vi "Big_LED_control.vi"() -> ()   [LabVIEW 2018]
uses:
  C:/Users/user/Desktop/LabVIEW/LED_CONTROL_big/LED_CONTROL_big_LED_ophir_ready/AT lib/AmateurStepperMotor.dll
  AT lib/AmateurStepperMotor.dll
  <instrlib>/niDMM/nidmm.llb/niDMM Function.ctl
  <instrlib>/niDMM/nidmm.llb/niDMM Resolution in Digits.ctl
  <instrlib>/niDCPower/nidcpower.llb/niDCPower Measurement Type.ctl
  <vilib>/Instr/_visa.llb/VISA Configure Serial Port (Instr).vi
  <instrlib>/niDMM/nidmm.llb/niDMM Configure Measurement Digits.vi
panel:
  in  "Tab Control 2":enum32{"Шаговик и офир", "Служебная область"}(tab)
  in  "milliseconds to wait":u32=1000
  in  "Go To":dbl
  out "Ophir 1 Char":dbl(graph)=0.060000000000000005
  in  "DecelerationTime, s":dbl
  in  "AccelerationTime, s":dbl
  in  "HoldOn":bool
  in  "Ophir 1 units":string(combo)="1000" caption="Units"
  out "Ophir 1 Over Range":bool caption="Over Range"
  out "Ophir 1 Optical Power":dbl=0.060000000000000005 caption="Power" format="%#_4g"
  out "Ophir 1 MAX":dbl=0.060000000000000005 caption="MAX" format="%#_5g"
  in  "Ophir 1 Clear":bool caption="Clear"
  in  "StepMultiplicationFactor":dbl=1.0
  in  "StepDivisor":i32(ring)=8 items=["D1"=1, "D2"=2, "D4"=4, "D8"=8, "D16"=16, "D32"=32]
  in  "Speed":dbl=1000.0
  in  "Погнали!":bool
  in  "Стоп GoTo":bool
  out "Готово":bool
  out "Position":dbl
  in  "Ophir 1 Info":u16(ring)=1 caption="Info" items=["Device : JUNO; s/n:903793", "Head : PD300R-3W   ; s/n:779628"]
  in  "new pos":dbl
  in  "set pos":bool
  out "Device Response":string="*\n"
  in  "Ophir 1 usb channel":i16 caption="usb channel"
  out "Ophir 1 dup Visa Session":refnum<visa-resource-name>="USB0::0x0BD3::0x0777::NI-VISA-40004::RAW" caption="dup Visa Session"
  in  "Ophir 1 Baud Rate (3:9600)":i16(ring)=3 caption="Baud Rate (3:9600)" items=["300", "1200", "4800", "9600", "19200", "38400"]
  out "Ophir 1 Real Optical Power":dbl=6e-05 format="%.6e"
  in  "Ophir 1 GPIB Address (10)":string="10" caption="GPIB Address (10)"
  in  "Ophir 1 Port Number (default 2)":i16=1 caption="Port Number (default 2)" min=0 max=20
  in  "Ophir 1 Select Communication Protocol":u16(ring) caption="Select Communication Protocol" items=["USB", "RS232", "GPIB"]
  out "Ophir 1 error out":errorcluster caption="error out"
  in  "Ophir 1 error in (no error)":errorcluster caption="error in (no error)"
  in  "Ophir 1 Wait":u32=100 caption="Wait"
  out "IsOpen":bool
  out "Ophir 1 Initialization":bool=TRUE caption="Initialization"
  in  "Tab Control":T1(tab)=enum."Служебная область"
  in  "POWER":bool
  in  "Стоп":bool=TRUE
  in  "Resource Name":refnum<k15>="PXI1Slot2" caption="Источник питания"
  in  "Амперметр":refnum<k15>="PXI1Slot4" caption="NI DMM 1"
  in  "V_MB, V":dbl=5.0 caption="voltage level" format="%_6p"
  in  "curlim_V_MB, A":dbl=0.3 caption="current limit" format="%_6p"
  out "curmes_V_MB, A":dbl=-0.001986406197333734 caption="measurement" format="%_6g"
  out "chart_0":dbl(graph)=-0.001986406197333734 caption="Waveform Chart 5"
  in  "voltlim_I_LED, V":dbl=0.01 caption="current limit" min=0.01 format="%_6p"
  in  "I_LED, A":dbl=2.000000000000001 caption="voltage level" format="%_6p"
  out "chart_1":dbl(graph)=9.464711192498274e-07 caption="Waveform Chart 5"
  out "voltmes_V_LED, A":dbl=9.464711192498274e-07 caption="measurement" format="%_6g"
  out "Current Char":dbl(graph)=0.008323229849338531
  in  "Arduino":refnum<visa-resource-name>="COM14"
  in  "Сегменты":bool[](array[boolean])=[FALSE, FALSE, FALSE, FALSE, FALSE, FALSE, FALSE, FALSE, FALSE, FALSE, FALSE, FALSE, FALSE, FALSE, FALSE, FALSE, FALSE, FALSE]
  in  "Вольтметр":refnum<k15>="PXI1Slot5" caption="NI DMM 1"
  out "Voltage Char":dbl(graph)=nan
  in  "Port Name":string="COM1" caption="Порт шаговика"
  in  "wave_lenght":string="600"
  in  "Промер":bool caption="Промер сегмента"
  in  "NI DMM 1 Voltage Range 4":string(combo)="-1" caption="Range"
  in  "NI DMM 1 units 4":string(combo)="1" caption="Units"
  out "Voltage":dbl=nan format="%_6g"
  in  "NI DMM 1 Current Range 3":string(combo)="1" caption="Range"
  in  "NI DMM 1 units 3":string(combo)="1000" caption="Units"
  out "Current":dbl=0.008323229849338531 format="%_6g"
  out "Разряд":dbl
  out "+/-":bool
  out "Power off":bool=TRUE
  in  "Command":string="Anode"
  in  "Записать":bool
  out "measure output file refnum":refnum<file>
  out "Voltage, V":dbl=nan caption="Measurement" format="%.5f"
  out "Current, A":dbl=8.323229849338531e-06 caption="Measurement" format="%.5f"
  out "Тип индикатора":string="Anode"
  out "chart_2":dbl(graph)=4.286668577189643e-07
  in  "V_RES, V":dbl caption="voltage level" format="%_6p"
  out "curmes_V_RES, A":dbl=4.286668577189643e-07 caption="measurement" format="%_6g"
  in  "curlim_V_RES, A":dbl=0.1 caption="current limit" min=0.01 format="%_6p"
  in  "measure path":path=path "D:/NI LabVIEW/MultiOpto/MultiOpto_1.2/Logs/SEL"
  out "Enum":enum16{"Exit", "4", "Промер", "2", "1"}(ring)
  out "№ об-ца":dbl
  out "Темп-ра":dbl
  out "Сегмент":string
  # "Шаговик"
  # "Офир"
  # "Шаговик"
  # "Офир"
  # "position - это значение абсолютное"
  # "j"
  # "c"
  # "d"
  # "e"
  # "g"
  # "h"
  # "a"
  # "b"
  # "f"
  # "k"
  # "L"
  # "m"
  # "n"
  # "p"
  # "dp"
  # "all"
  # "V_MB 5 В\nогрничение 300 м\n\nV_LED 2,1 В\nограничение 200 м"
  # "единицы мА\nrange 1 А"
  # "1. каждый сегмент включаем по отдельности, резистором постраиваем ток до 10 мА\n2. напряжение V_LED при этом не меняется\n3. в такоом положении промеряем сегменты по отдельности\n4. для промера всего индикатора сразу подстраиваем напряжение при неизменном положении резисторов\n5. ток всех индикаторов = ток одного сегмента (10 мА) * число сегментов (15)\n6. добиваемся этого увеличением V_LED"
  # "единицы В\nrange AUTO"
  # "регклировка суммарного тока через индикатор"
  # "24.063\n\n     I          U\n20 мА  1.3 В\n20 мА  1.4 В\n 7 мА   1.15 В"
  # "24.064\n\n     I          U\n10 мА  2 В\n10 мА  2.15 В\n 7 мА   1.9 В"
  # "автоматизировать подбор напряжения по известному максимальному напряжению и току. ОС по току сегмента"
  # "Р1:  +25°C\nР2:  - 60°C\nР3:  +85°C"
  # "регулировать ток в зависимости от температуры.\nс ростом температуры растет ток.\nпид-регулятор??"
  # "0. ввести номер образца\n1. включить нужный сегмент\n2. ввести его в поле справа\n3. вести температуру в поле слева\n4. нажать кнопку \"промер сегмента\""
  # "\"опрашивать кнопки не чаще, чем раз в секунду. сейчас кликать можно чаще, они загорятся, но ничего не произойдет\""
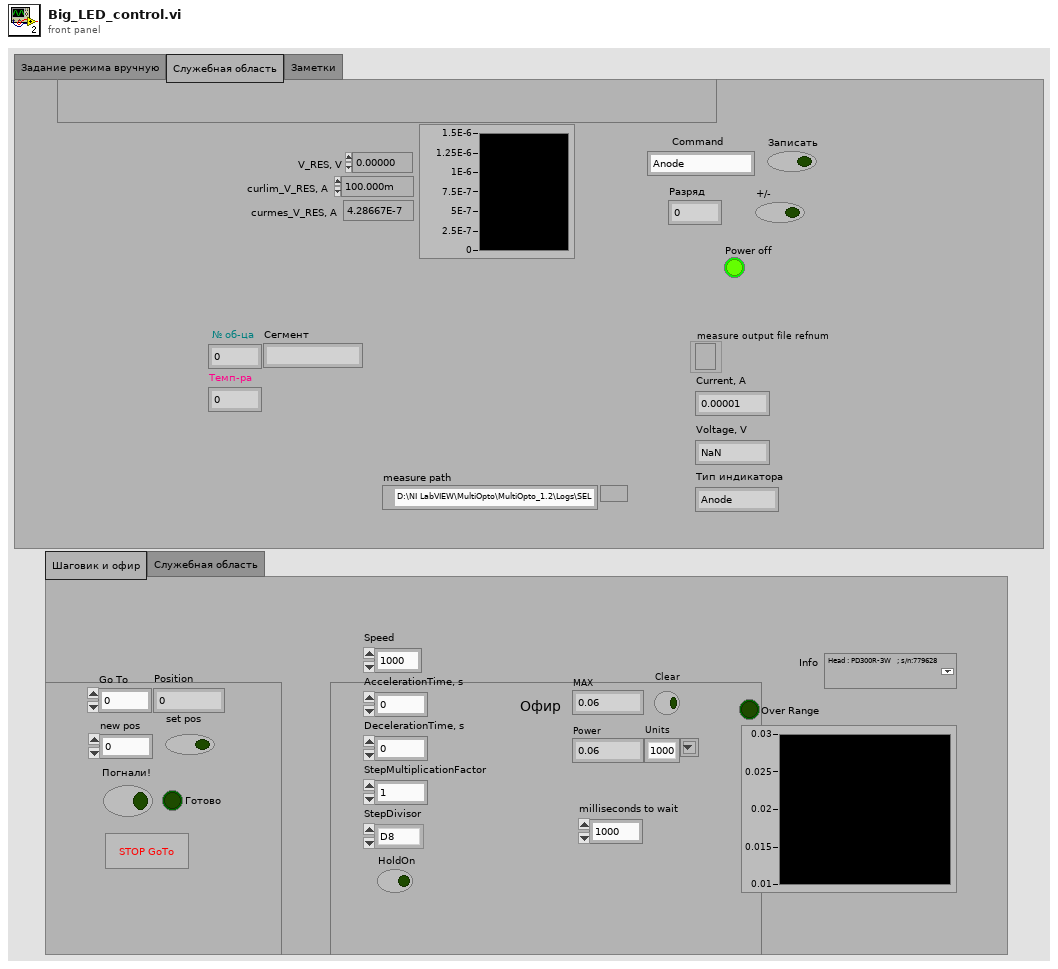
[diagram p1: front panel]
types:
  T1 = enum32{"Задание режима вручную", "Служебная область", "Заметки"}
  T2 = enum16{"open", "replace", "create", "open or create", "replace or create", "replace or create with confirmation"}
  T3 = typedef "niDCPower Measurement Type.ctl" = i32
  T4 = typedef "niDMM Function.ctl" = enum16{"DC Volts", "AC Volts", "DC Current", "AC Current", "2-wire Resistance", "4-wire Resistance", "Diode", "Frequency", "Period", "AC Volts DC Coupled", "Capacitance", "Inductance", "Temperature"}
  T5 = typedef "niDMM Resolution in Digits.ctl" = dbl
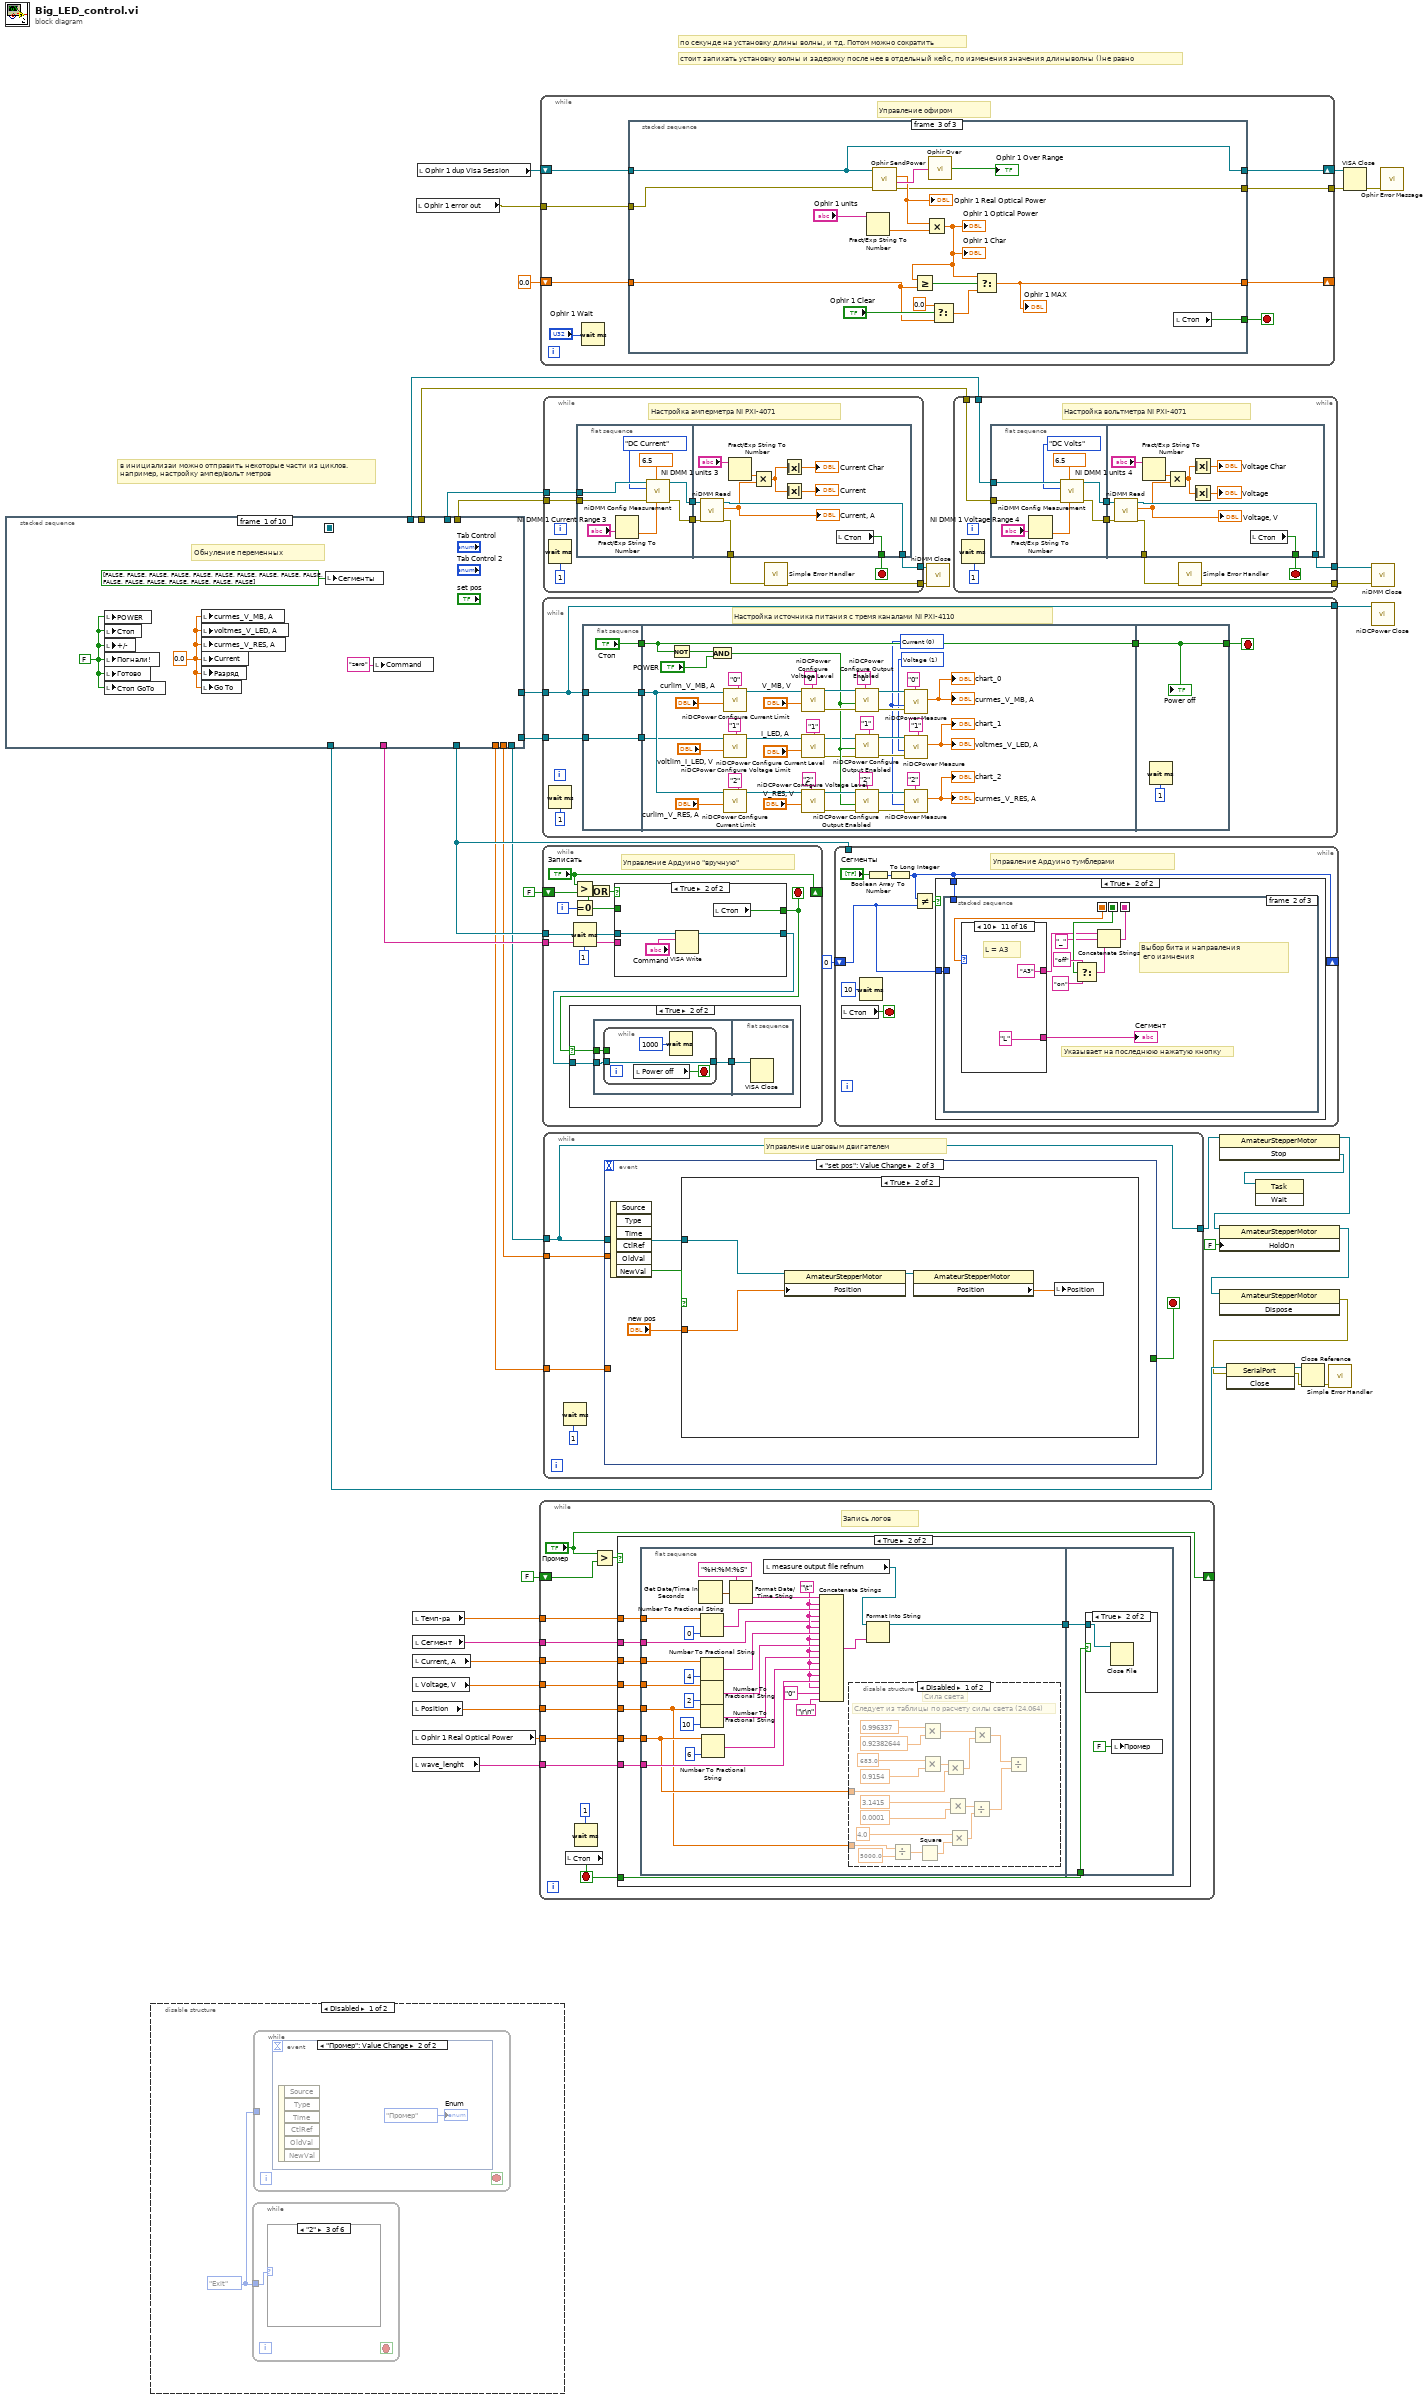
[diagram p0: block diagram]
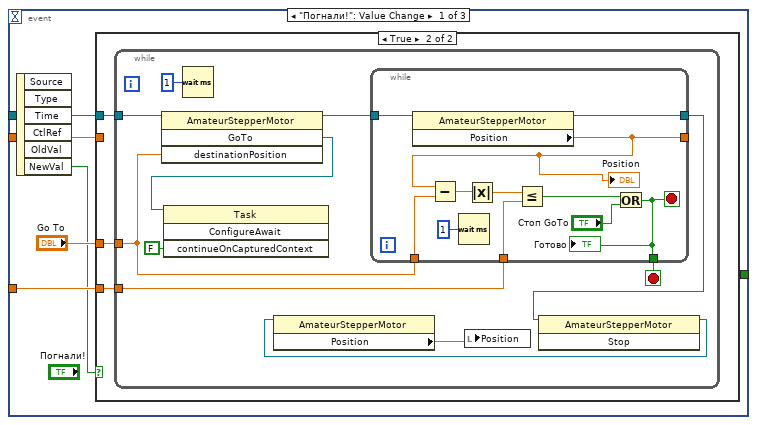
[diagram p2: hidden frame]
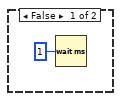
[diagram p3: hidden frame]
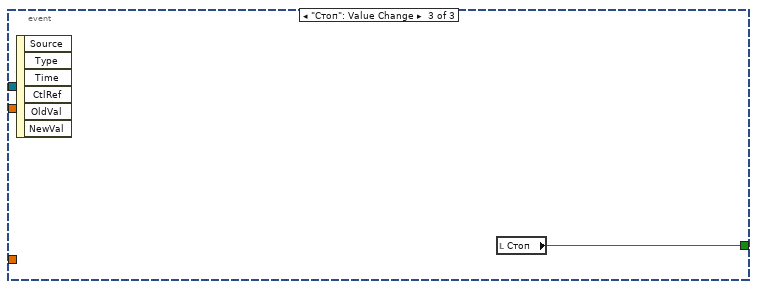
[diagram p5: hidden frame]
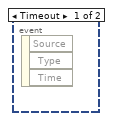
[diagram p11: hidden frame]
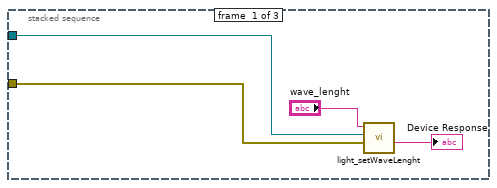
[diagram p16: hidden frame]
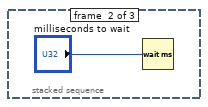
[diagram p17: hidden frame]
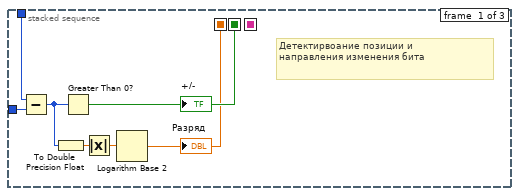
[diagram p19: hidden frame]
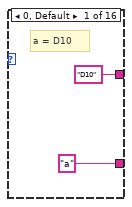
[diagram p20: hidden frame]
diagram:
  # "в инициализаи можно отправить некоторые части из циклов.\nнапример, настройку ампер/вольт метров"
  # "стоит запихать установку волны и задержку после нее в отдельный кейс, по изменения значения длиныволны ()не равно"
  # "по секунде на установку длины волны, и тд. Потом можно сократить"
  n1 = stacked-sequence {
    seq-local: [_ _ _ _ _ _ w97 _ _ _] -> [_ _ _ _ _ _ _ w106 _ _]
    tunnel: [_ _ _ w59 _ _ _ _ _ _] -> w30
    tunnel: [_ w49 _ _ _ _ _ _ _ _] -> w42
    tunnel: [_ w48 _ _ _ _ _ _ _ _] -> w41
    tunnel: [_ _ _ _ w64 _ _ _ _ _] -> w38
    tunnel: [_ _ _ _ _ _ _ _ _ w146] -> w37
    tunnel: [_ _ w52 _ _ _ _ _ _ _] -> w36
    tunnel: [_ _ w51 _ _ _ _ _ _ _] -> w35
    tunnel: [_ _ _ _ _ _ _ w109 _ _] -> w29
    tunnel: [_ _ _ _ _ _ _ w107 _ _] -> w27
    tunnel: [_ _ _ _ _ _ _ w108 _ _] -> w28
    tunnel: [_ _ _ _ _ _ w87 _ _ _] -> w21
    tunnel: [_ _ _ w53 _ _ _ _ _ _] -> w4
    frame #0 {
      w43 = 0.0 ("currentmes_2")
      w44 = FALSE ("Стоп")
      # "Обнуление переменных"
      n2 = local write "POWER"(w44) -> ()
      n3 = local write "Стоп"(w44) -> ()
      n4 = local write "+/-"(w44) -> ()
      n5 = local write "Погнали!"(w44) -> ()
      n6 = local write "Готово"(w44) -> ()
      n7 = local write "Стоп GoTo"(w44) -> ()
      n8 = local write "curmes_V_MB, A"(w43) -> ()
      n9 = local write "voltmes_V_LED, A"(w43) -> ()
      n10 = local write "curmes_V_RES, A"(w43) -> ()
      n11 = local write "Current"(w43) -> ()
      n12 = local write "Разряд"(w43) -> ()
      n13 = local write "Go To"(w43) -> ()
      n14 = local write "Сегменты"(bool[] [FALSE, FALSE, FALSE, FALSE, FALSE, FALSE, FALSE, FALSE, FALSE, FALSE, FALSE, FALSE, FALSE, FALSE, FALSE, FALSE, FALSE, FALSE] ("Сегменты")) -> ()
      n15 = local write "Command"("zero" ("Command 2")) -> ()
    }
    frame #1 {
      # "Инициализация амперметра"
      n16 = call <instrlib>:"niDMM Initialize.vi"("Instrument Descriptor"="Амперметр") -> ("error out"=w49:errorcluster, "instrument handle out"=w48:refnum<k15>)  [unwired: 9 in]
    }
    frame #2 {
      # "Инициализация вольтметра"
      n17 = call <instrlib>:"niDMM Initialize.vi"("Instrument Descriptor"="Вольтметр") -> ("error out"=w51:errorcluster, "instrument handle out"=w52:refnum<k15>)  [unwired: 9 in]
    }
    frame #3 {
      # "Инициализация источника питания"
      n18 = call <instrlib>:"niDCPower Initialize.vi"("resource name"="Resource Name") -> ("error out"=w61:errorcluster, "instrument handle out"=w62:refnum<k15>)  [unwired: 3 in, 6 out]
      n19 = call <instrlib>:"niDCPower Initialize.vi"("resource name"="Resource Name") -> ("error out"=w54:errorcluster, "instrument handle out"=w55:refnum<k15>)  [unwired: 3 in, 6 out]
      n20 = call <instrlib>:"niDCPower Configure Current Level.vi"("error in (no error)"=w54, "current level"=0.0, "channel name"="1", "instrument handle"=w55) -> ("instrument handle out"=w53:refnum<k15>)  [unwired: 6 in, 1 out]
      n21 = call <instrlib>:"niDCPower Configure Voltage Level.vi"("error in (no error)"=w61, "voltage level"=0.0, "channel name"="0,2", "instrument handle"=w62) -> ("instrument handle out"=w59:refnum<k15>)  [unwired: 6 in, 1 out]
    }
    frame #4 {
      # "Инициализация Ардуино"
      n22 = call-poly "VISA Configure Serial Port"("VISA resource name"="Arduino", "baud rate (9600)"=u32 9600) -> ("VISA resource name out"=w64:refnum<visa-resource-name>)  [unwired: 12 in, 1 out]
    }
    frame #5 {
      # "Инициализация офира"
      n23 = call "Ophir InitCom.vi"("GPIB Address (default 10)"="Ophir 1 GPIB Address (10)", "Communication (default USB 0)"="Ophir 1 Select Communication Protocol", "USB Channel number (default 0)"="Ophir 1 usb channel", "Port Number (default 2)"="Ophir 1 Port Number (default 2)", "error in (no error)"="Ophir 1 error in (no error)", "Baud Rate (3:9600)"="Ophir 1 Baud Rate (3:9600)") -> ("dup Visa Session"=w73:refnum<visa-resource-name>, "error out"=w72:errorcluster)  [unwired: 1 out]
      n24 = call "Ophir InstrInfo.vi"("Visa Session"=w73, "error in (no error)"=w72) -> ("dup Visa Session"=w85:refnum<visa-resource-name>, "Instrument Info"=w67:string, "error out"=w83:errorcluster)
      n25 = call "Ophir HeadInfo.vi"("Visa Session"=w85, "error in (no error)"=w83) -> ("error out"=w82:errorcluster, "dup Visa Session"=w84:refnum<visa-resource-name>, "Head Info"=w81:string)  [unwired: 6 out]
      n26 = call "Ophir InfoStrings.vi"("error in (no error)"=w82, "Head Info"=w81, "Instrument Info"=w67) -> ("error out"=w80:errorcluster, "Strings Array"=w79:string[])
      n27 = property on="Ophir 1 Info" class="Ring (strict)"("Strings []"=w79) -> ()  [unwired: 2 in, 2 out]
      n28 = call "Ophir ConfigDevice.vi"("Visa Session"=w84, "Measure Choice (0:Power)"=u16 0, "error in (no error)"=w80) -> ("dup Visa Session"=→"Ophir 1 dup Visa Session":refnum<visa-resource-name>, "OK ?"=→"Ophir 1 Initialization":bool, "error out"=→"Ophir 1 error out":errorcluster)  [unwired: 1 out]
    }
    frame #6 {
      w91 = 100 ("WriteTimeout")
      w96 = 1 items=["None", "One", "Two", "OnePointFive"] ("stopBits")
      w93 = 0 items=["None", "Odd", "Even", "Mark", "Space"] ("parity")
      # "убрали открытие порта. шаговик его и так сам откроет"
      # "Инициализация шаговика ч.1"
      n29 = constructor class="SerialPort"("portName"="Port Name", "baudRate"=57600, "parity"=w93, "dataBits"=8, "stopBits"=w96) -> (reference out=w90:refnum<k24>, error out=w89:errorcluster)  [unwired: 3 in, 6 out]
      n30 = property class="SerialPort"(reference=w90, error in=w89, "WriteTimeout"=w91, "ReadTimeout"=w91) -> (reference out=w87:refnum<k24>)  [unwired: 1 out]
      n31 = constructor class="AmateurStepperMotor"("serialPort"=w87) -> (reference out=w97:refnum<k24>, error out=w88:errorcluster)  [unwired: 3 in, 2 out]
      n32 = flat-sequence {
        tunnel: w88 -> [_]
        tunnel: w87 -> [w99]
        frame #0 {
          n33 = property class="SerialPort"(reference=w99) -> ("IsOpen"=→"IsOpen":bool)  [unwired: 1 in, 2 out]
        }
      }
    }
    frame #7 {
      # "стоит допустить изменение\nтих параметров в цикле, а не только \nпри инициализации"
      # "это те самые 50 шагов за мм"
      # "Инициализация шаговика ч.2"
      n34 = property class="AmateurStepperMotor"(reference=w106, "Speed"="Speed", "StepDivisor"="StepDivisor", "StepMultiplicationFactor"="StepMultiplicationFactor", "AccelerationTime"="AccelerationTime, s", "DecelerationTime"="DecelerationTime, s", "HoldOn"="HoldOn") -> (reference out=w109:refnum<k24>, "Position"=w107:dbl, "PositioningPrecision"=w108:dbl)  [unwired: 1 in, 1 out]
    }
    frame #8 {
      w115 = "\t"
      # "Инициализация логов"
      n35 = local read "№ об-ца"() -> (w111:dbl)
      n36 = Number To Fractional String(number=w111, precision (6)=i16 0) -> (F-format string=w112:string)  [unwired: 2 in]
      n37 = Get Date/Time In Seconds() -> (seconds since 1Jan1904=w133:timestamp)
      n38 = Build Path(base path="measure path", name or relative path=w112) -> (appended path=w129:path)
      n39 = call <vilib>:"Check if File or Folder Exists.vi"("path"=w129) -> ("file or folder exists?"=w130:bool, "dup path"=w131:path)  [unwired: 8 in, 1 out]
      n40 = Format Date/Time String(time format string (%c)="MES %d %m %y %H.%M.%S", seconds (now)=w133) -> (date/time string=w134:string)  [unwired: 1 in]
      n41 = case shown="False" w130 {
        tunnel: w131 -> [w142 w143]
        tunnel: [w141 w143] -> w132
        frame False {
          n42 = Create Folder(path (use dialog)=w142) -> (created path=w141:path)  [unwired: 2 in, 2 out]
        }
        frame True {
        }
      }
      n43 = Concatenate Strings(w134, ".xls" ("string")) -> (w135:string)
      n44 = Build Path(base path=w132, name or relative path=w135) -> (appended path=w136:path)
      n45 = Open/Create/Replace File(file path (use dialog)=w136, operation (0:open)=T2."open or create", access (0:read/write)=enum16{"read/write", "read-only", "write-only"}."read/write") -> (refnum out=w137:refnum<file>)  [unwired: 3 in, 2 out]
      n46 = Set File Position(refnum=w137, from (0:start)=enum16{"start", "end", "current"}."end") -> (refnum out=w139:refnum<file>)  [unwired: 2 in, 1 out]
      n47 = Format Into String(initial string=w139, "Time" ("string"), w115, "Temperature, C" ("string"), w115, "Segment" ("string"), w115, "Current, mA" ("string"), w115, "Voltage, V" ("input 7"), w115, "Distance, m" ("string"), w115, "Power, W " ("string"), w115, "Wavelenght, nm" ("input 17"), w115, "Candlepower, kd" ("string"), "\r\n") -> (resulting string=→"measure output file refnum":refnum<file>)  [unwired: 2 in, 1 out]
    }
    frame #9 {
      # "Begin VI: ОК или ОА?"
      n48 = call "Begin.vi"() -> ("Темп-ра"=→"Темп-ра":dbl, "№ об-ца"=→"№ об-ца":dbl, "String"=w146:string)  [unwired: 6 in]
      "Тип индикатора" <- w146
      n49 = local write "Command"(w146) -> ()
    }
  }
  n50 = disable-structure shown="Disabled" {
    frame Disabled {
      w147 = enum16{"Exit", "4", "Промер", "2", "1"}."Exit"
      n51 = while {
        tunnel: w147 -> [w148]
        stop <- _ stop-if-true
        n52 = case shown="\"2\"" w148 {
          frame "Exit", Default {
          }
          frame "4" {
          }
          frame "2" {
          }
          frame "2" {
          }
          frame "1" {
          }
          frame "Промер" {
          }
        }
      }
      n53 = while {
        tunnel: w147 -> [_]
        stop <- _ stop-if-true
        n54 = event shown="[1] \"Промер\": Value Change" {
          selector: _ -> [_ _]
          dyn-events: _ -> [_ _]
          timeout: _ -> [_ _]
          event Timeout {
            n55 = event-data() -> ()  [unwired: 1 in, 3 out]
          }
          event "Промер": Value Change {
            n56 = event-data() -> ()  [unwired: 1 in, 6 out]
            "Enum" <- enum16{"Exit", "4", "Промер", "2", "1"}."Промер" ("Enum")
          }
        }
      }
    }
    frame Enabled {
    }
  }
  n57 = local read "Темп-ра"() -> (w2:dbl)
  n58 = local read "Сегмент"() -> (w1:string)
  n59 = local read "Current, A"() -> (w20:dbl)
  n60 = local read "Voltage, V"() -> (w19:dbl)
  n61 = local read "Position"() -> (w18:dbl)
  n62 = local read "Ophir 1 Real Optical Power"() -> (w17:dbl)
  n63 = local read "wave_lenght"() -> (w16:string)
  n64 = local read "Ophir 1 error out"() -> (w25:errorcluster)
  n65 = local read "Ophir 1 dup Visa Session"() -> (w26:refnum<visa-resource-name>)
  n66 = while {
    tunnel: w20 -> [w161]
    tunnel: w19 -> [w160]
    tunnel: w18 -> [w159]
    tunnel: w17 -> [w158]
    tunnel: w16 -> [w157]
    shift-right: ["Промер"] -> _
    shift-left: FALSE ("Промер сегмента") -> [w154]
    tunnel: w2 -> [w151]
    tunnel: w1 -> [w150]
    stop <- w152 stop-if-true
    # "Запиcь логов"
    n67 = local read "Стоп"() -> (w152:bool)
    n68 = Wait (ms)(milliseconds to wait=u32 1) -> ()  [unwired: 1 out]
    n69 = Greater?(x="Промер", y=w154) -> (0:w155:bool)
    n70 = case shown="True" w155 {
      tunnel: w161 -> [_ w170]
      tunnel: w160 -> [_ w169]
      tunnel: w159 -> [_ w166]
      tunnel: w158 -> [_ w167]
      tunnel: w157 -> [_ w168]
      tunnel: w152 -> [_ w164]
      tunnel: w151 -> [_ w163]
      tunnel: w150 -> [_ w162]
      frame False {
      }
      frame True {
        n71 = flat-sequence {
          tunnel: w170 -> [w188]
          tunnel: w169 -> [w187]
          tunnel: w168 -> [w185]
          tunnel: w167 -> [w184]
          tunnel: w166 -> [w183]
          tunnel: [w178] -> w165
          tunnel: w163 -> [w177]
          tunnel: w162 -> [w171]
          tunnel: w165 -> [w218]
          tunnel: w164 -> [w217]
          frame #0 {
            w173 = "\t"
            n72 = Get Date/Time In Seconds() -> (seconds since 1Jan1904=w196:timestamp)
            n73 = Number To Fractional String(number=w177, precision (6)=i16 0) -> (F-format string=w175:string)  [unwired: 2 in]
            n74 = Number To Fractional String(number=w188, precision (6)=i16 4) -> (F-format string=w191:string)  [unwired: 2 in]
            n75 = Number To Fractional String(number=w187, precision (6)=i16 2) -> (F-format string=w190:string)  [unwired: 2 in]
            n76 = Number To Fractional String(number=w183, precision (6)=i16 10) -> (F-format string=w189:string)  [unwired: 2 in]
            n77 = Number To Fractional String(number=w184, precision (6)=i16 6) -> (F-format string=w186:string)  [unwired: 2 in]
            n78 = Format Date/Time String(time format string (%c)="%H:%M:%S", seconds (now)=w196) -> (date/time string=w194:string)  [unwired: 1 in]
            n79 = local read "measure output file refnum"() -> (w192:refnum<file>)
            n80 = Concatenate Strings(w194, w173, w175, w173, w171, w173, w191, w173, w190, w173, w189, w173, w186, w173, w185, w173, "0" ("string"), "\r\n") -> (w193:string)
            n81 = disable-structure shown="Disabled" {
              disable-tunnel: w184 -> [w208 _]
              disable-tunnel: w183 -> [w198 _]
              frame Disabled {
                # "Сила света"
                # "Следует из таблицы по расчету силы света (24.064)"
                n82 = Divide(x=w198, y=5000.0) -> (x/y=w200:dbl)
                n83 = Square(x=w200) -> (x^2=w199:dbl)
                n84 = Multiply(x=0.996337, y=0.92382644) -> (x*y=w213:dbl)
                n85 = Multiply(x=683.0, y=0.9154) -> (x*y=w209:dbl)
                n86 = Multiply(x=w209, y=w208) -> (x*y=w207:dbl)
                n87 = Multiply(x=3.1415, y=0.0001) -> (x*y=w203:dbl)
                n88 = Multiply(x=4.0, y=w199) -> (x*y=w202:dbl)
                n89 = Divide(x=w203, y=w202) -> (x/y=w204:dbl)
                n90 = Multiply(x=w213, y=w207) -> (x*y=w212:dbl)
                n91 = Divide(x=w212, y=w204) -> ()  [unwired: 1 out]
              }
              frame Enabled {
              }
            }
            n92 = Format Into String(initial string=w192, w193) -> (resulting string=w178:refnum<file>)  [unwired: 2 in, 1 out]
          }
          frame #1 {
            n93 = case shown="True" w217 {
              tunnel: w218 -> [_ w219]
              frame False {
              }
              frame True {
                n94 = Close File(refnum=w219) -> ()  [unwired: 1 in, 2 out]
              }
            }
            n95 = local write "Промер"(FALSE ("Промер")) -> ()
          }
        }
      }
    }
  }
  n96 = while {
    tunnel: w25 -> [w226]
    shift-right: [w222] -> _
    shift-left: 0.0 ("t") -> [w225]
    shift-right: [w223] -> w14
    shift-left: w26 -> [w227]
    tunnel: [w221] -> w13
    stop <- w220 stop-if-true
    # "Управление офиром"
    n97 = Wait (ms)(milliseconds to wait="Ophir 1 Wait") -> ()  [unwired: 1 out]
    n98 = stacked-sequence {
      tunnel: w227 -> [w231 _ w234]
      tunnel: w226 -> [w230 _ w236]
      tunnel: w225 -> [_ _ w237]
      tunnel: [_ _ w234] -> w223
      tunnel: [_ _ w238] -> w222
      tunnel: [_ _ w235] -> w221
      tunnel: [_ _ w233] -> w220
      frame #0 {
        n99 = call "light_setWaveLenght.vi"("error in (no error)"=w230, "Visa Session"=w231, "wave_lenght"="wave_lenght") -> ("Device Response"=→"Device Response":string)  [unwired: 6 in, 2 out]
      }
      frame #1 {
        n100 = Wait (ms)(milliseconds to wait="milliseconds to wait") -> ()  [unwired: 1 out]
      }
      frame #2 {
        n101 = Fract/Exp String To Number(string="Ophir 1 units") -> (number=w241:dbl)  [unwired: 3 in, 1 out]
        n102 = call "Ophir SendPower.vi"("Visa Session"=w234, "error in (no error)"=w236) -> ("Value Number"=w240:dbl, "Value String"=w247:string, "error out"=w235:errorcluster)  [unwired: 1 out]
        "Ophir 1 Real Optical Power" <- w240
        n103 = Multiply(x=w240, y=w241) -> (x*y=w244:dbl)
        "Ophir 1 Char" <- w244
        "Ophir 1 Optical Power" <- w244
        n104 = Greater Or Equal?(x=w244, y=w237) -> (x >= y?=w245:bool)
        n105 = call "Ophir Over.vi"("Value String"=w247) -> ("Overrange"=→"Ophir 1 Over Range":bool)
        n106 = Select(t=0.0, s="Ophir 1 Clear", f=w237) -> (s? t:f=w243:dbl)
        n107 = Select(t=w244, s=w245, f=w243) -> (s? t:f=w238:dbl)
        "Ophir 1 MAX" <- w238
        n108 = local read "Стоп"() -> (w233:bool)
      }
    }
  }
  n109 = while {
    tunnel: w30 -> [w253]
    tunnel: [w253] -> w39
    tunnel: w4 -> [w250]
    stop <- w249 stop-if-true
    # "Настройка источника питания с тремя каналами NI PXI-4110"
    n110 = Wait (ms)(milliseconds to wait=u32 1) -> ()  [unwired: 1 out]
    n111 = flat-sequence {
      tunnel: w253 -> [w259]
      tunnel: [w259] -> w255
      tunnel: ["Стоп"] -> w254
      tunnel: [w257] -> w251
      tunnel: w250 -> [w257]
      tunnel: w255 -> [w276]
      tunnel: w254 -> [w303]
      tunnel: [w303] -> w252
      tunnel: w251 -> [w267]
      tunnel: [w305] -> w249
      tunnel: w252 -> [w305]
      frame #0 {
      }
      frame #1 {
        w260 = T3 1 items=["Current", "Voltage"] ("measurement type")
        w275 = T3 0 items=["Current", "Voltage"] ("measurement type")
        n112 = Not(x=w303) -> (.not. x?=w302:bool)
        n113 = And(x=w302, y="POWER") -> (x .and. y?=w271:bool)
        n114 = call <instrlib>:"niDCPower Configure Current Limit.vi"("current limit"="curlim_V_MB, A", "channel name"="0", "instrument handle"=w276) -> ("instrument handle out"=w293:refnum<k15>)  [unwired: 7 in, 1 out]
        n115 = call <instrlib>:"niDCPower Configure Voltage Limit.vi"("voltage limit"="voltlim_I_LED, V", "channel name"="1", "instrument handle"=w267) -> ("instrument handle out"=w264:refnum<k15>)  [unwired: 7 in, 1 out]
        n116 = call <instrlib>:"niDCPower Configure Current Limit.vi"("current limit"="curlim_V_RES, A", "channel name"="2", "instrument handle"=w276) -> ("instrument handle out"=w292:refnum<k15>)  [unwired: 7 in, 1 out]
        n117 = call <instrlib>:"niDCPower Configure Voltage Level.vi"("voltage level"="V_MB, V", "channel name"="0", "instrument handle"=w293) -> ("error out"=w298:errorcluster, "instrument handle out"=w295:refnum<k15>)  [unwired: 7 in]
        n118 = call <instrlib>:"niDCPower Configure Current Level.vi"("current level"="I_LED, A", "channel name"="1", "instrument handle"=w264) -> ("error out"=w262:errorcluster, "instrument handle out"=w265:refnum<k15>)  [unwired: 7 in]
        n119 = call <instrlib>:"niDCPower Configure Voltage Level.vi"("voltage level"="V_RES, V", "channel name"="2", "instrument handle"=w292) -> ("error out"=w297:errorcluster, "instrument handle out"=w296:refnum<k15>)  [unwired: 7 in]
        n120 = call <instrlib>:"niDCPower Configure Output Enabled.vi"("error in (no error)"=w298, "output enabled"=w271, "channel name"="0", "instrument handle"=w295) -> ("error out"=w288:errorcluster, "instrument handle out"=w289:refnum<k15>)  [unwired: 6 in]
        n121 = call <instrlib>:"niDCPower Configure Output Enabled.vi"("error in (no error)"=w262, "output enabled"=w271, "channel name"="1", "instrument handle"=w265) -> ("error out"=w300:errorcluster, "instrument handle out"=w299:refnum<k15>)  [unwired: 6 in]
        n122 = call <instrlib>:"niDCPower Configure Output Enabled.vi"("error in (no error)"=w297, "output enabled"=w271, "channel name"="2", "instrument handle"=w296) -> ("error out"=w287:errorcluster, "instrument handle out"=w286:refnum<k15>)  [unwired: 6 in]
        n123 = call <instrlib>:"niDCPower Measure.vi"("error in (no error)"=w288, "measurement type"=w275, "channel name"="0", "instrument handle"=w289) -> ("measurement"=→"curmes_V_MB, A" →"chart_0":dbl)  [unwired: 5 in, 2 out]
        n124 = call <instrlib>:"niDCPower Measure.vi"("error in (no error)"=w300, "measurement type"=w260, "channel name"="1", "instrument handle"=w299) -> ("measurement"=→"chart_1" →"voltmes_V_LED, A":dbl)  [unwired: 5 in, 2 out]
        n125 = call <instrlib>:"niDCPower Measure.vi"("error in (no error)"=w287, "measurement type"=w275, "channel name"="2", "instrument handle"=w286) -> ("measurement"=→"curmes_V_RES, A" →"chart_2":dbl)  [unwired: 5 in, 2 out]
      }
      frame #2 {
        n126 = Wait (ms)(milliseconds to wait=u32 1) -> ()  [unwired: 1 out]
        "Power off" <- w305
      }
    }
  }
  n127 = while {
    tunnel: w38 -> [w313]
    shift-right: ["Записать"] -> _
    shift-left: FALSE ("Записать") -> [w315]
    tunnel: w37 -> [w311]
    i -> [w312]
    stop <- w306 stop-if-true
    # "Управление Ардуино \"вручную\""
    n128 = Greater?(x="Записать", y=w315) -> (0:w309:bool)
    n129 = Equal To 0?(x=w312) -> (x = 0?=w308:bool)
    n130 = Wait (ms)(milliseconds to wait=u32 1) -> ()  [unwired: 1 out]
    n131 = Or(x=w309, y=w308) -> (x .or. y?=w310:bool)
    n132 = case shown="True" w310 {
      tunnel: w313 -> [w327 w332]
      tunnel: [w328 w331] -> w306
      tunnel: w311 -> [_ _]
      tunnel: w308 -> [_ _]
      tunnel: [w327 w329] -> w307
      frame False {
        n133 = local read "Стоп"() -> (w328:bool)
      }
      frame True {
        n134 = VISA Write(VISA resource name=w332, write buffer="Command") -> (VISA resource name out=w329:refnum<visa-resource-name>)  [unwired: 1 in, 2 out]
        n135 = local read "Стоп"() -> (w331:bool)
      }
    }
    n136 = case shown="True" w306 {
      selector: w306 -> [_ w317]
      tunnel: w307 -> [_ w319]
      frame False {
      }
      frame True {
        n137 = flat-sequence {
          tunnel: w319 -> [w322]
          tunnel: [w321] -> w318
          tunnel: w317 -> [w320]
          tunnel: w318 -> [w326]
          frame #0 {
            n138 = while {
              tunnel: w322 -> [w325]
              tunnel: [w325] -> w321
              tunnel: w320 -> [_]
              stop <- w323 stop-if-true
              n139 = local read "Power off"() -> (w323:bool)
              n140 = Wait (ms)(milliseconds to wait=u32 1000) -> ()  [unwired: 1 out]
            }
          }
          frame #1 {
            n141 = VISA Close(VISA resource name=w326) -> ()  [unwired: 1 in, 1 out]
          }
        }
      }
    }
  }
  n142 = while {
    tunnel: [w339] -> w31
    tunnel: w41 -> [w337]
    tunnel: w42 -> [w336]
    tunnel: [w333] -> w32
    stop <- w335 stop-if-true
    # "Настройка амперметра NI PXI-4071"
    n143 = Wait (ms)(milliseconds to wait=u32 1) -> ()  [unwired: 1 out]
    n144 = flat-sequence {
      tunnel: [w346] -> w341
      tunnel: w337 -> [w344]
      tunnel: w336 -> [w348]
      tunnel: [w345] -> w340
      tunnel: w341 -> [w357]
      tunnel: w340 -> [w360]
      tunnel: [w356] -> w335
      tunnel: [w355] -> w333
      tunnel: [w354] -> w334
      frame #0 {
        w342 = T5 6.5 items=["3 1/2"=3.5, "4 1/2"=4.5, "5 1/2"=5.5, "6 1/2"=6.5, "7 1/2"=7.5] ("Resolution in Digits")
        n145 = Fract/Exp String To Number(string="NI DMM 1 Current Range 3") -> (number=w347:dbl)  [unwired: 3 in, 1 out]
        n146 = call-poly <instrlib>:"niDMM Config Measurement.vi"("Range"=w347, "Resolution in Digits"=w342, "error in (no error)"=w348, "Function"=niDMM_Function."DC Current" ("Measurement Type"), "instrument handle"=w344) -> ("error out"=w345:errorcluster, "instrument handle out"=w346:refnum<k15>)  [unwired: 5 in]
      }
      frame #1 {
        n147 = call <instrlib>:"niDMM Read.vi"("error in (no error)"=w360, "instrument handle"=w357) -> ("error out"=w354:errorcluster, "Measurement"=w350:dbl, "instrument handle out"=w355:refnum<k15>)  [unwired: 7 in]
        "Current, A" <- w350
        n148 = Fract/Exp String To Number(string="NI DMM 1 units 3") -> (number=w358:dbl)  [unwired: 3 in, 1 out]
        n149 = Multiply(x=w358, y=w350) -> (x*y=w351:dbl)
        n150 = Absolute Value(x=w351) -> (abs(x)=→"Current Char":dbl)
        n151 = Absolute Value(x=w351) -> (abs(x)=→"Current":dbl)
        n152 = local read "Стоп"() -> (w356:bool)
      }
    }
    n153 = call <vilib>:"Simple Error Handler.vi"("error in (no error)"=w334) -> ("error out"=w339:errorcluster)  [unwired: 1 in, 7 out]
  }
  n154 = while {
    tunnel: w29 -> [w362]
    tunnel: w28 -> [w364]
    tunnel: [w362] -> w3
    tunnel: w27 -> [w365]
    stop <- w361 stop-if-true
    # "Управление шаговым двигателем"
    n155 = Wait (ms)(milliseconds to wait=u32 1) -> ()  [unwired: 1 out]
    n156 = event shown="[1] \"set pos\": Value Change" {
      selector: _ -> [_ _ _]
      dyn-events: _ -> [_ _ _]
      timeout: _ -> [_ _ _]
      tunnel: w362 -> [w370 w398 _]
      tunnel: w365 -> [w369 _ _]
      tunnel: w364 -> [w368 _ _]
      tunnel: [_ _ w404] -> w361
      event "Погнали!": Value Change {
        n157 = event-data() -> ("NewVal"=w366:bool)  [unwired: 1 in, 5 out]
        n158 = case shown="True" w366 {
          tunnel: "Go To" -> [_ w374]
          tunnel: w370 -> [_ w373]
          tunnel: w369 -> [_ _]
          tunnel: w368 -> [_ w372]
          frame False {
            n159 = Wait (ms)(milliseconds to wait=u32 1) -> ()  [unwired: 1 out]
          }
          frame True {
            n160 = while {
              tunnel: w374 -> [w381]
              tunnel: w373 -> [w382]
              tunnel: w372 -> [w384]
              stop <- w385 stop-if-true
              n161 = invoke class="AmateurStepperMotor" method="GoTo"(reference=w382, "destinationPosition"=w381) -> (reference out=w377:refnum<k24>, "GoTo"=w380:refnum<k24>)  [unwired: 2 in, 2 out]
              n162 = invoke class="Task" method="ConfigureAwait"(reference=w380, "continueOnCapturedContext"=FALSE) -> ()  [unwired: 2 in, 4 out]
              n163 = Wait (ms)(milliseconds to wait=u32 1) -> ()  [unwired: 1 out]
              n164 = while {
                tunnel: [w386] -> _
                tunnel: [w388] -> w378
                tunnel: [w390] -> w385
                tunnel: w381 -> [w395]
                tunnel: w384 -> [w393]
                tunnel: w377 -> [w387]
                stop <- w390 stop-if-true
                n165 = property class="AmateurStepperMotor"(reference=w387) -> (reference out=w388:refnum<k24>, "Position"=w386:dbl)  [unwired: 1 in, 1 out]
                "Position" <- w386
                n166 = Subtract(x=w386, y=w395) -> (x-y=w396:dbl)
                n167 = Wait (ms)(milliseconds to wait=u32 1) -> ()  [unwired: 1 out]
                n168 = Absolute Value(x=w396) -> (abs(x)=w394:dbl)
                n169 = Less Or Equal?(x=w394, y=w393) -> (x <= y?=w392:bool)
                n170 = Or(x=w392, y="Стоп GoTo") -> (x .or. y?=w390:bool)
                "Готово" <- w390
              }
              n171 = invoke class="AmateurStepperMotor" method="Stop"(reference=w378) -> (reference out=w376:refnum<k24>)  [unwired: 2 in, 2 out]
              n172 = property class="AmateurStepperMotor"(reference=w376) -> ("Position"=w375:dbl)  [unwired: 1 in, 2 out]
              n173 = local write "Position"(w375) -> ()
            }
          }
        }
      }
      event "set pos": Value Change {
        n174 = event-data() -> ("NewVal"=w399:bool)  [unwired: 1 in, 5 out]
        n175 = case shown="True" w399 {
          tunnel: w398 -> [_ w403]
          tunnel: "new pos" -> [_ w402]
          frame False {
          }
          frame True {
            n176 = property class="AmateurStepperMotor"(reference=w403, "Position"=w402) -> (reference out=w401:refnum<k24>)  [unwired: 1 in, 1 out]
            n177 = property class="AmateurStepperMotor"(reference=w401) -> ("Position"=w400:dbl)  [unwired: 1 in, 2 out]
            n178 = local write "Position"(w400) -> ()
          }
        }
      }
      event "Стоп": Value Change {
        n179 = event-data() -> ()  [unwired: 1 in, 6 out]
        n180 = local read "Стоп"() -> (w404:bool)
      }
    }
  }
  n181 = while {
    shift-right: [w407] -> _
    shift-left: 0 -> [w408]
    tunnel: w38 -> [_]
    stop <- w411 stop-if-true
    # "Управление Ардуино тумблерами"
    n182 = local read "Стоп"() -> (w411:bool)
    n183 = Wait (ms)(milliseconds to wait=u32 10 ("millisecond timer value")) -> ()  [unwired: 1 out]
    n184 = Boolean Array To Number(Boolean array="Сегменты") -> (number=w406:u32)
    n185 = To Long Integer(number=w406) -> (32bit integer=w407:i32)
    n186 = Not Equal?(x=w407, y=w408) -> (x != y?=w409:bool)
    n187 = case shown="True" w409 {
      tunnel: w407 -> [_ w412]
      tunnel: w408 -> [_ w413]
      frame False {
      }
      frame True {
        n188 = stacked-sequence {
          seq-local: [w416 _ _] -> [_ w427 _]
          seq-local: [w414 _ _] -> [_ w422 _]
          seq-local: [_ w423 _] -> [_ _ w463]
          tunnel: w412 -> [w418 _ _]
          tunnel: w413 -> [w417 _ _]
          frame #0 {
            # "Детектирвоание позиции и\nнаправления изменения бита"
            n189 = Subtract(x=w418, y=w417) -> (x-y=w419:i32)
            n190 = To Double Precision Float(number=w419) -> (double precision float=w420:dbl)
            n191 = Greater Than 0?(x=w419) -> (x > 0?=w416:bool)
            "+/-" <- w416
            n192 = Absolute Value(x=w420) -> (abs(x)=w415:dbl)
            n193 = Logarithm Base 2(1:w415) -> (0:w414:dbl)
            "Разряд" <- w414
          }
          frame #1 {
            # "Указывает на последнюю нажатую кнопку"
            # "Выбор бита и направления\n его измнения"
            n194 = case shown="10" w422 {
              tunnel: ["D10" "D9" "D5" "D8" "D11" "D12" "A1" "D4" "A5" "A4" "A3" "A2" "A0" "D13" "D3" "All"] -> w425
              tunnel: ["a" "b" "c" "d" "e" "f" "g" "h" "j" "k" "L" "m" "n" "p" "dp" "All"] -> w421
              frame 0, Default {
                # "a = D10"
              }
              frame 1 {
                # "b = D9"
              }
              frame 2 {
                # "c = D5"
              }
              frame 3 {
                # "d = D8"
              }
              frame 4 {
                # "e = D11"
              }
              frame 5 {
                # "f = D12"
              }
              frame 6 {
                # "g = A1"
              }
              frame 7 {
                # "h = D4"
              }
              frame 8 {
                # "j = A5"
              }
              frame 9 {
                # "k = A4"
              }
              frame 10 {
                # "L = A3"
              }
              frame 11 {
                # "m = A2"
              }
              frame 12 {
                # "n = A0"
              }
              frame 13 {
                # "p = D13"
              }
              frame 14 {
                # "dp = D3"
              }
              frame 15 {
              }
            }
            "Сегмент" <- w421
            n195 = Select(t="off", s=w427, f="on") -> (s? t:f=w424:string)
            n196 = Concatenate Strings(w425, "_" ("string"), w424) -> (w423:string)
          }
          frame #2 {
            # "Передача команды в Ардуино"
            n197 = Equal?(x=w463, y="All_off") -> (x = y?=w466:bool)
            n198 = Equal?(x=w463, y="All_on") -> (x = y?=w464:bool)
            n199 = case shown="True" w466 {
              frame False {
              }
              frame True {
                n200 = local write "Сегменты"(bool[] [TRUE, TRUE, TRUE, TRUE, TRUE, TRUE, TRUE, TRUE, TRUE, TRUE, TRUE, TRUE, TRUE, TRUE, TRUE, TRUE] ("Сегменты")) -> ()
              }
            }
            n201 = case shown="True" w464 {
              frame False {
              }
              frame True {
                n202 = local write "Сегменты"(bool[] [FALSE, FALSE, FALSE, FALSE, FALSE, FALSE, FALSE, FALSE, FALSE, FALSE, FALSE, FALSE, FALSE, FALSE, FALSE, FALSE] ("Сегменты")) -> ()
              }
            }
            n203 = stacked-sequence {
              tunnel: w463 -> [w469 _ _]
              frame #0 {
                n204 = local write "Command"(w469) -> ()
              }
              frame #1 {
                n205 = local write "Записать"(TRUE ("Записать")) -> ()
                n206 = Wait (ms)(milliseconds to wait=u32 1000) -> ()  [unwired: 1 out]
              }
              frame #2 {
                n207 = local write "Записать"(FALSE ("Записать")) -> ()
                n208 = Wait (ms)(milliseconds to wait=u32 1000) -> ()  [unwired: 1 out]
              }
            }
          }
        }
      }
    }
  }
  n209 = call <instrlib>:"niDMM Close.vi"("error in (no error)"=w31, "instrument handle"=w32) -> ()  [unwired: 9 in, 1 out]
  n210 = while {
    tunnel: [w480] -> w33
    tunnel: w36 -> [w478]
    tunnel: w35 -> [w477]
    tunnel: [w474] -> w34
    stop <- w476 stop-if-true
    # "Настройка вольтметра NI PXI-4071"
    n211 = Wait (ms)(milliseconds to wait=u32 1) -> ()  [unwired: 1 out]
    n212 = flat-sequence {
      tunnel: [w487] -> w482
      tunnel: w478 -> [w485]
      tunnel: w477 -> [w489]
      tunnel: [w486] -> w481
      tunnel: w482 -> [w498]
      tunnel: w481 -> [w501]
      tunnel: [w497] -> w476
      tunnel: [w496] -> w474
      tunnel: [w495] -> w475
      frame #0 {
        w483 = T5 6.5 items=["3 1/2"=3.5, "4 1/2"=4.5, "5 1/2"=5.5, "6 1/2"=6.5, "7 1/2"=7.5] ("Resolution in Digits")
        n213 = Fract/Exp String To Number(string="NI DMM 1 Voltage Range 4") -> (number=w488:dbl)  [unwired: 3 in, 1 out]
        n214 = call-poly <instrlib>:"niDMM Config Measurement.vi"("Range"=w488, "Resolution in Digits"=w483, "error in (no error)"=w489, "Function"=niDMM_Function."DC Volts" ("Measurement Type"), "instrument handle"=w485) -> ("error out"=w486:errorcluster, "instrument handle out"=w487:refnum<k15>)  [unwired: 5 in]
      }
      frame #1 {
        n215 = call <instrlib>:"niDMM Read.vi"("error in (no error)"=w501, "instrument handle"=w498) -> ("error out"=w495:errorcluster, "Measurement"=w493:dbl, "instrument handle out"=w496:refnum<k15>)  [unwired: 7 in]
        "Voltage, V" <- w493
        n216 = Fract/Exp String To Number(string="NI DMM 1 units 4") -> (number=w499:dbl)  [unwired: 3 in, 1 out]
        n217 = Multiply(x=w499, y=w493) -> (x*y=w491:dbl)
        n218 = Absolute Value(x=w491) -> (abs(x)=→"Voltage Char":dbl)
        n219 = Absolute Value(x=w491) -> (abs(x)=→"Voltage":dbl)
        n220 = local read "Стоп"() -> (w497:bool)
      }
    }
    n221 = call <vilib>:"Simple Error Handler.vi"("error in (no error)"=w475) -> ("error out"=w480:errorcluster)  [unwired: 1 in, 7 out]
  }
  n222 = invoke class="AmateurStepperMotor" method="Stop"(reference=w3) -> (reference out=w10:refnum<k24>, "Stop"=w11:refnum<k24>)  [unwired: 2 in, 1 out]
  n223 = property class="AmateurStepperMotor"(reference=w10, "HoldOn"=FALSE) -> (reference out=w9:refnum<k24>)  [unwired: 1 in, 1 out]
  n224 = invoke class="AmateurStepperMotor" method="Dispose"(reference=w9) -> (error out=w6:errorcluster)  [unwired: 2 in, 2 out]
  n225 = invoke class="SerialPort" method="Close"(reference=w21, error in=w6) -> (reference out=w5:refnum<k24>, error out=w7:errorcluster)  [unwired: 1 in, 1 out]
  n226 = invoke class="Task" method="Wait"(reference=w11) -> ()  [unwired: 2 in, 3 out]
  n227 = Close Reference(reference=w5, error in (no error)=w7) -> (error out=w8:errorcluster)
  n228 = call <vilib>:"Simple Error Handler.vi"("error in (no error)"=w8) -> ()  [unwired: 1 in, 8 out]
  n229 = VISA Close(VISA resource name=w14, error in (no error)=w13) -> (error out=w23:errorcluster)
  n230 = call <instrlib>:"niDMM Close.vi"("error in (no error)"=w33, "instrument handle"=w34) -> ()  [unwired: 9 in, 1 out]
  n231 = call <instrlib>:"niDCPower Close.vi"("instrument handle"=w39) -> ()  [unwired: 10 in, 1 out]
  n232 = call "Ophir Error Message.vi"("error in (no error)"=w23) -> ()  [unwired: 3 in, 4 out]
